vi "Install Linux Image.vi"(8 "error in (no error)":errorcluster, 11 "Selected Targets":T1[](array[typedef]) {"Primary NIC"."IP Address Request Mode" items=["Static"=1, "DHCP/Link-Local"=2, "Link-Local Only"=4, "DHCP Only"=8]}) -> (0 "error out":errorcluster, 1 "Cancelled":bool)   [LabVIEW 2020]
uses:
  Controls/Installation Internal Variables.ctl
  Controls/Target Information.ctl
  Controls/Target Network Settings.ctl
  Controls/System Credentials.ctl
  Controls/Installation Notifiers.ctl
  Controls/Deployment Status Data Type.ctl
  Controls/Deployment Progress Data Type.ctl
  Controls/FP Control Functions.ctl
panel:
  out "Stop Updates":bool
  in  "Start Installation Process":bool
  in  "Stop":bool
  in  "Internal Variables":T4 {"Targets"."Primary NIC"."IP Address Request Mode" items=["Static"=1, "DHCP/Link-Local"=2, "Link-Local Only"=4, "DHCP Only"=8]}
  out "Targets":i32(listbox)
  in  "Close":bool
  # "Targets"
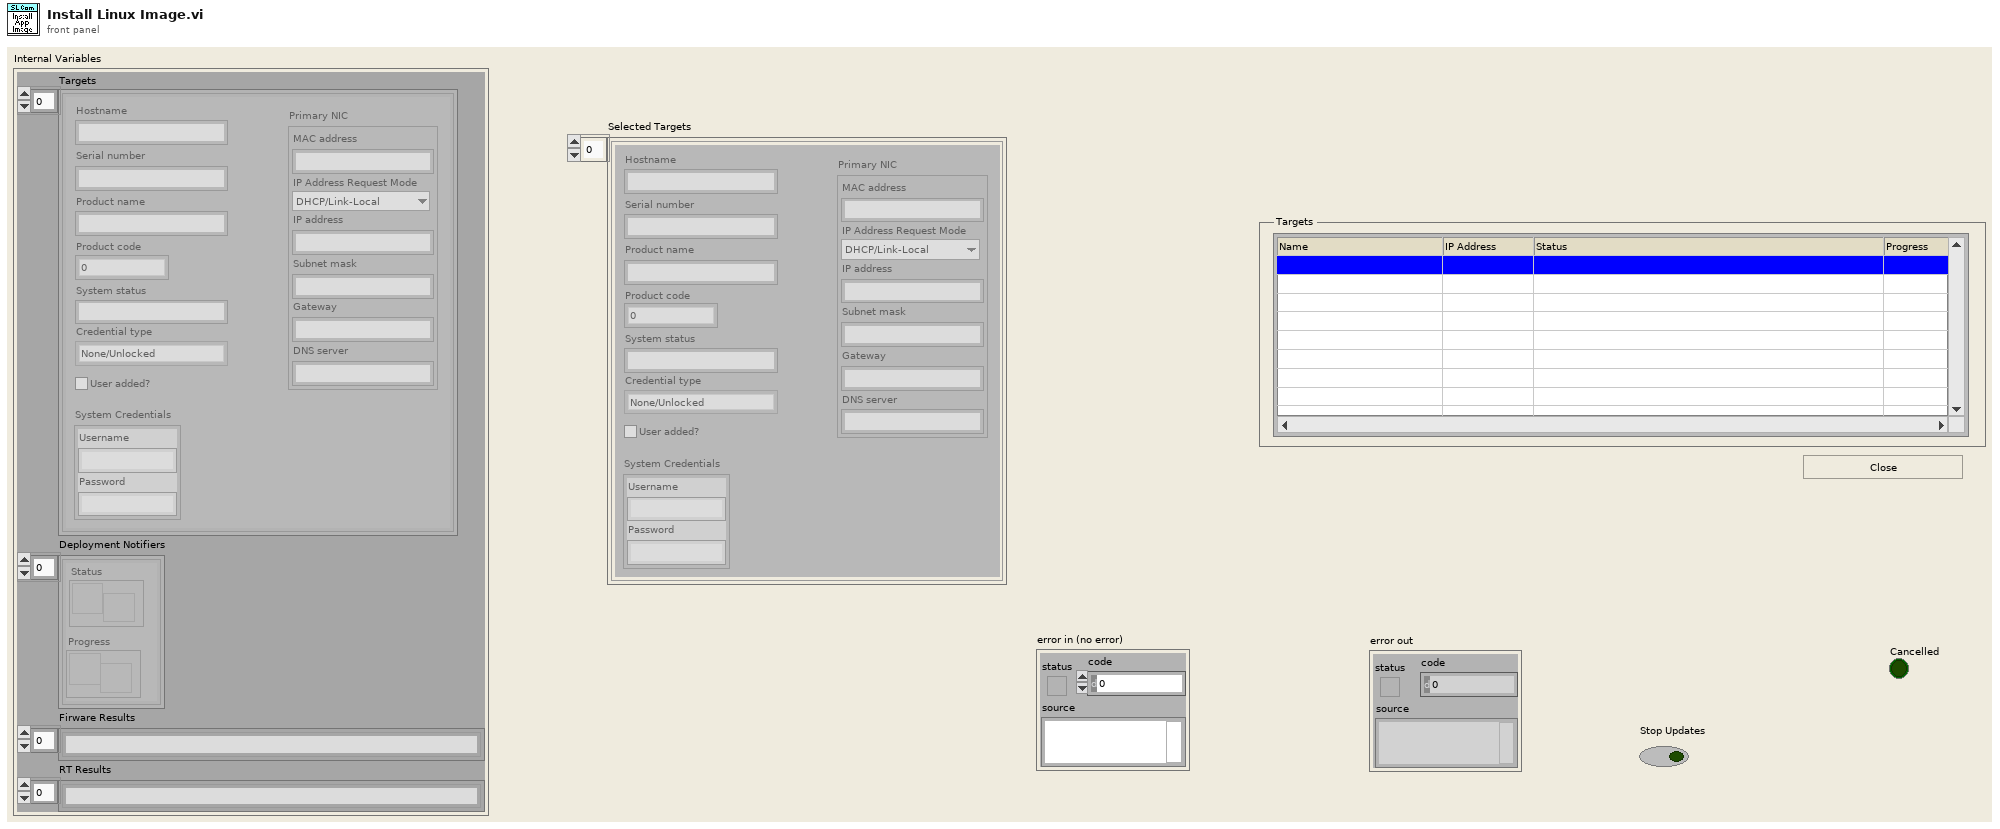
[diagram p1: front panel]
types:
  T1 = typedef "Target Information.ctl" = cluster{"Hostname":string, "Serial number":string, "Product name":string, "Product code":i32, "System status":string, "Credential type":enum16{"None/Unlocked", "FTP Password", "NIAuth Credentials"}, "User added?":bool, "Primary NIC":T2, "System Credentials":T3}
  T2 = typedef "Target Network Settings.ctl" = cluster{"MAC address":string, "IP Address Request Mode":i32, "IP address":string, "Subnet mask":string, "Gateway":string, "DNS server":string}
  T3 = typedef "System Credentials.ctl" = cluster{"Username":string, "Password":string}
  T4 = typedef "Installation Internal Variables.ctl" = cluster{"Targets":T1[], "Deployment Notifiers":T5[], "Firware Results":string[], "RT Results":string[]}
  T5 = typedef "Installation Notifiers.ctl" = cluster{"Status":refnum<notifier>, "Progress":refnum<notifier>}
  T6 = enum8{"Enabled", "Disabled", "Disabled and Grayed Out"}
  T7 = typedef "Deployment Progress Data Type.ctl" = i8
  T8 = typedef "Deployment Status Data Type.ctl" = string
  T9 = typedef "FP Control Functions.ctl" = enum16{"Open", "Close", "Bring To Front", "Center"}
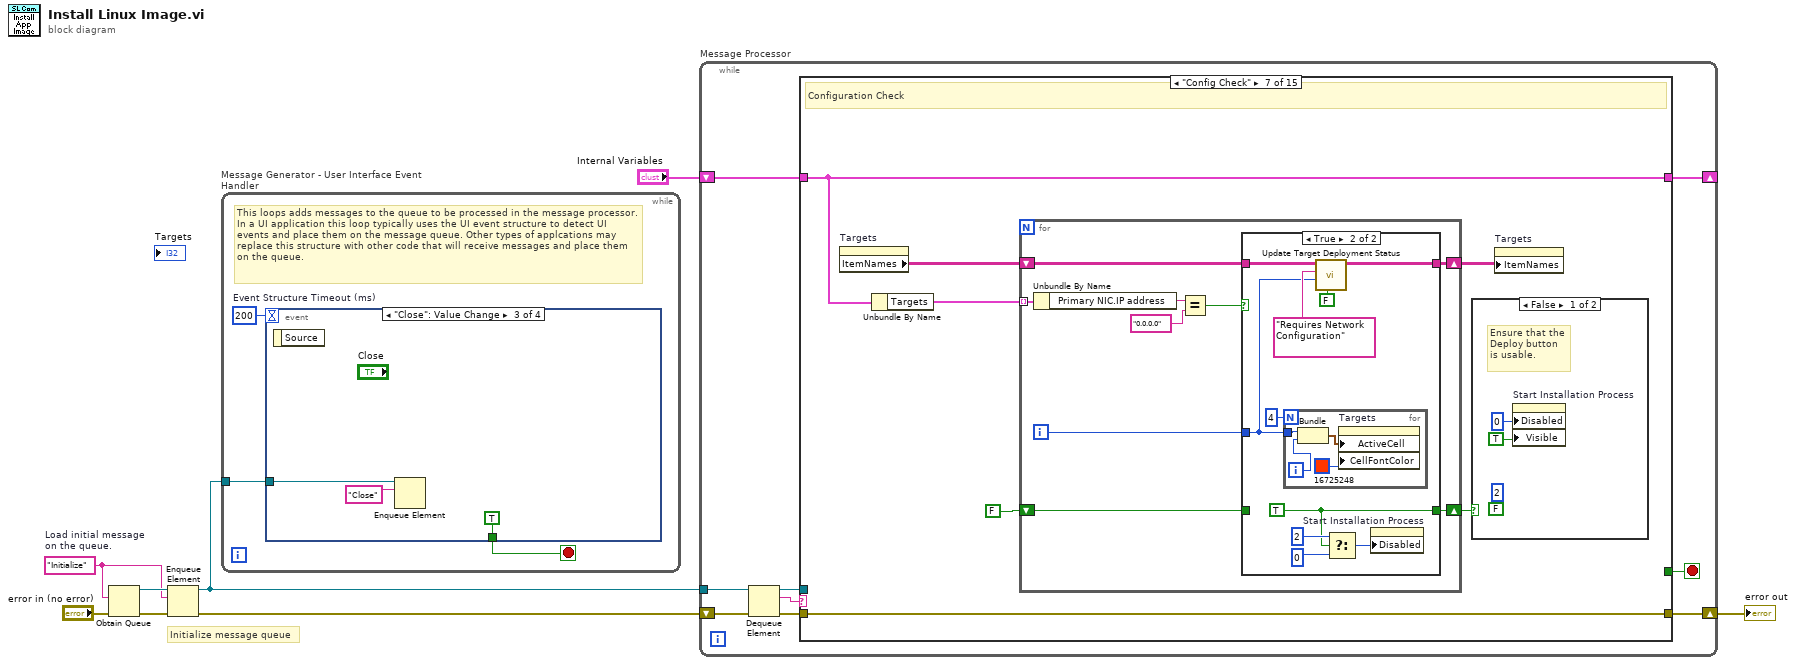
[diagram p0: block diagram]
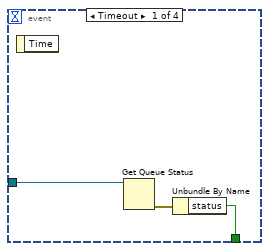
[diagram p2: hidden frame]
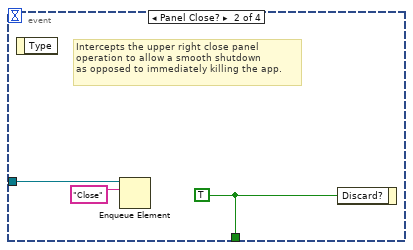
[diagram p3: hidden frame]
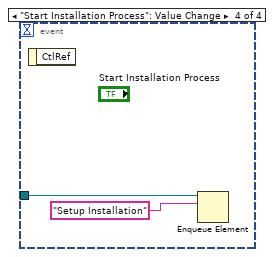
[diagram p4: hidden frame]
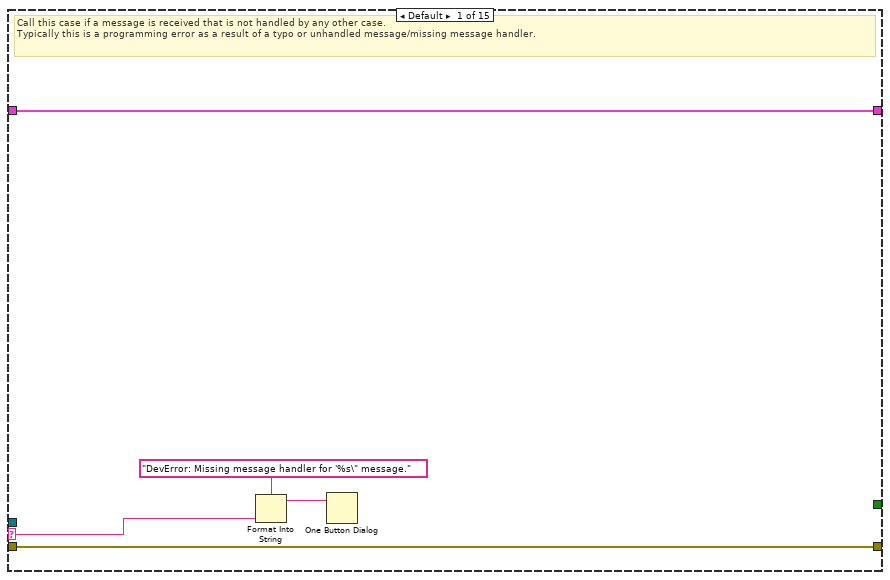
[diagram p5: hidden frame]
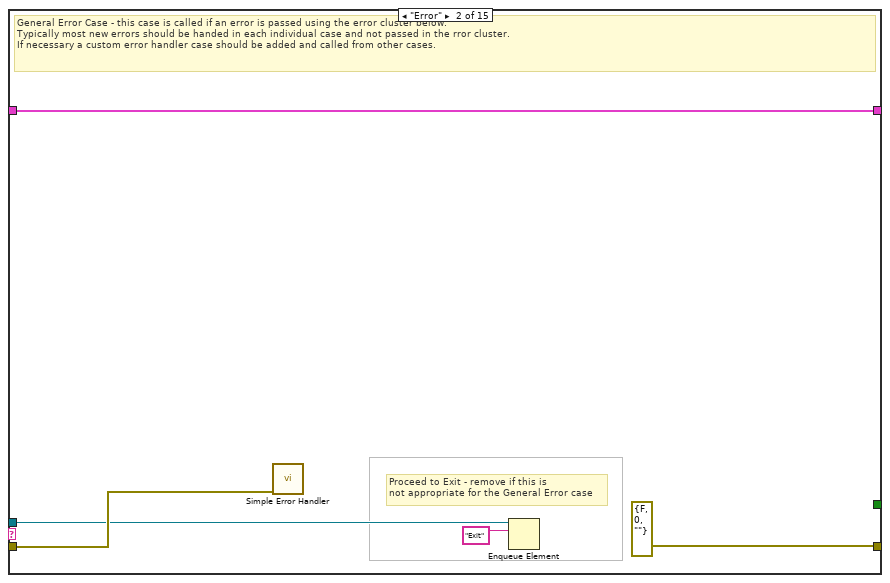
[diagram p6: hidden frame]
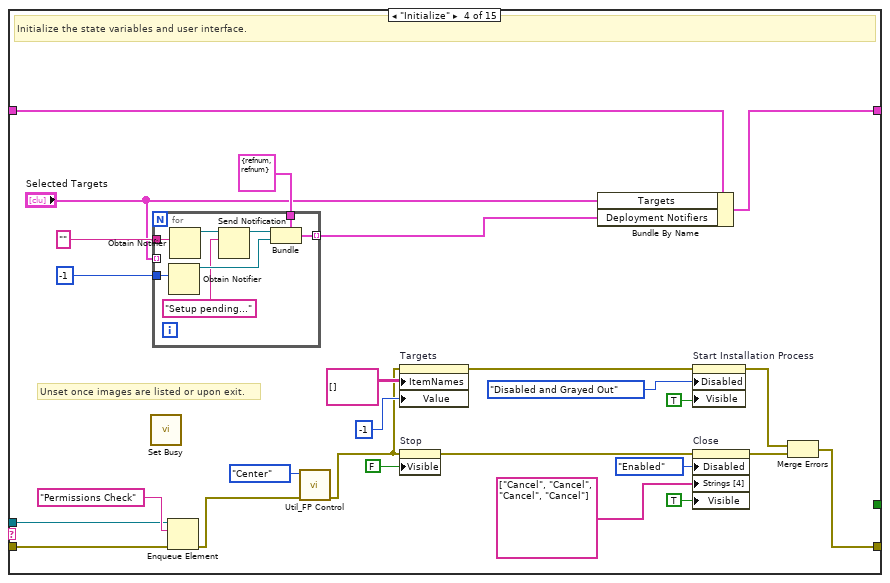
[diagram p8: hidden frame]
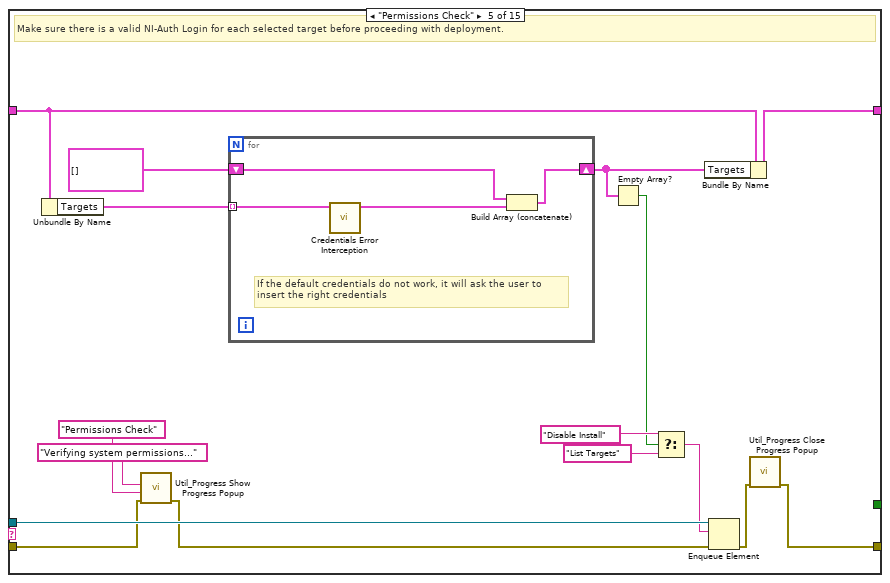
[diagram p9: hidden frame]
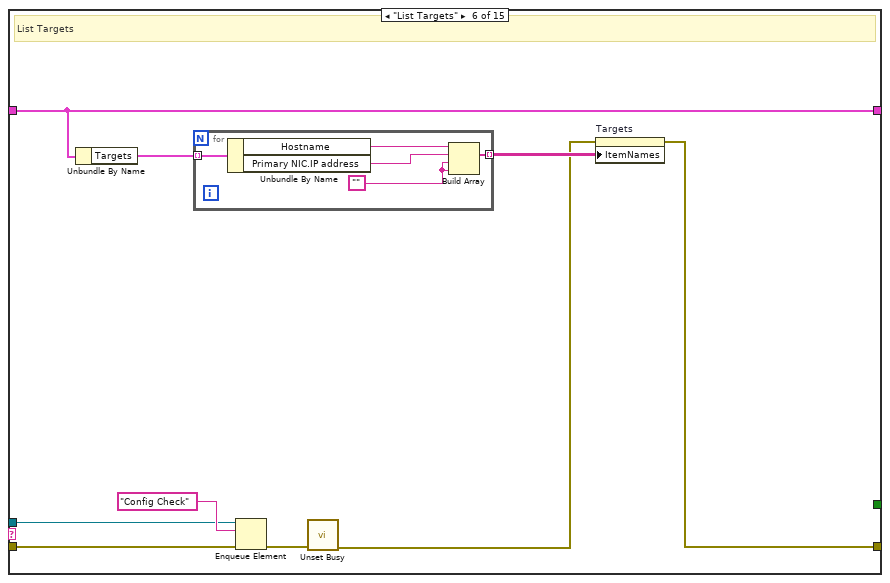
[diagram p10: hidden frame]
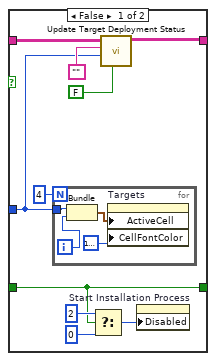
[diagram p12: hidden frame]
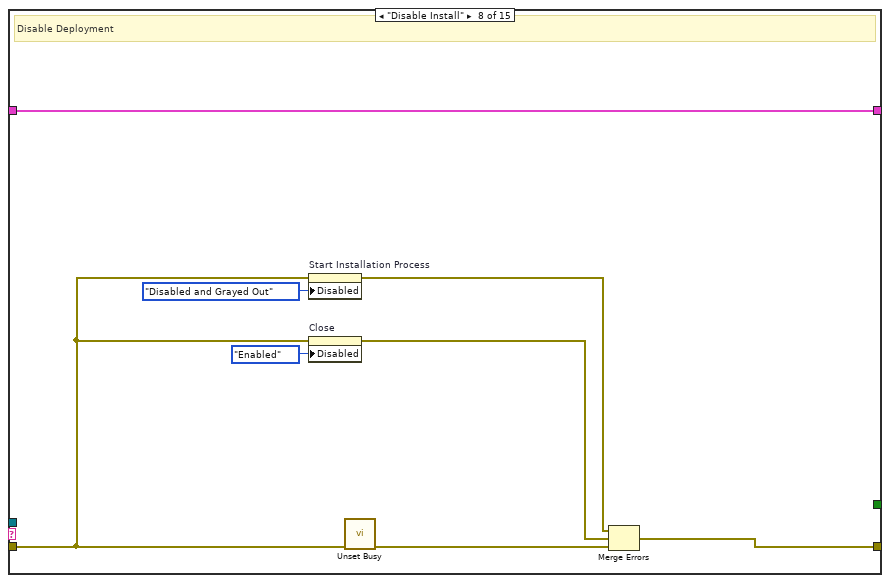
[diagram p13: hidden frame]
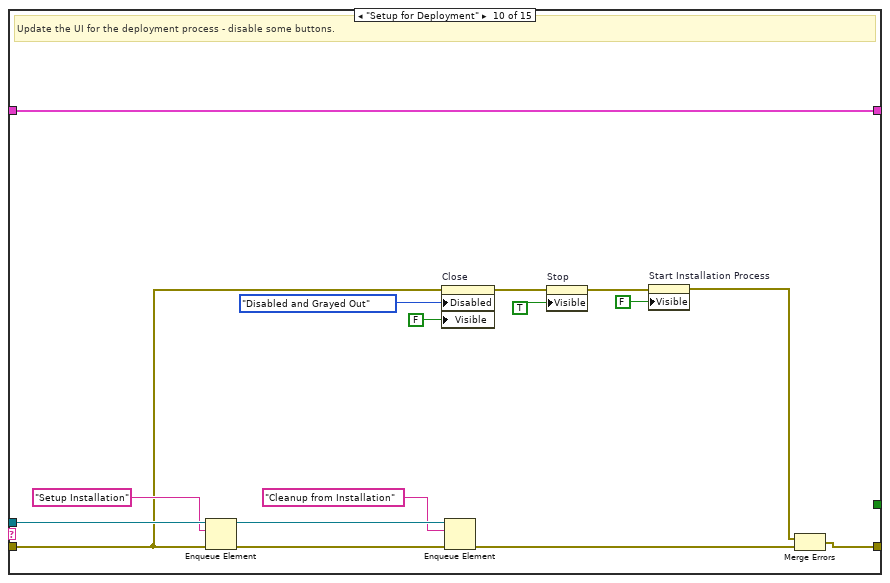
[diagram p15: hidden frame]
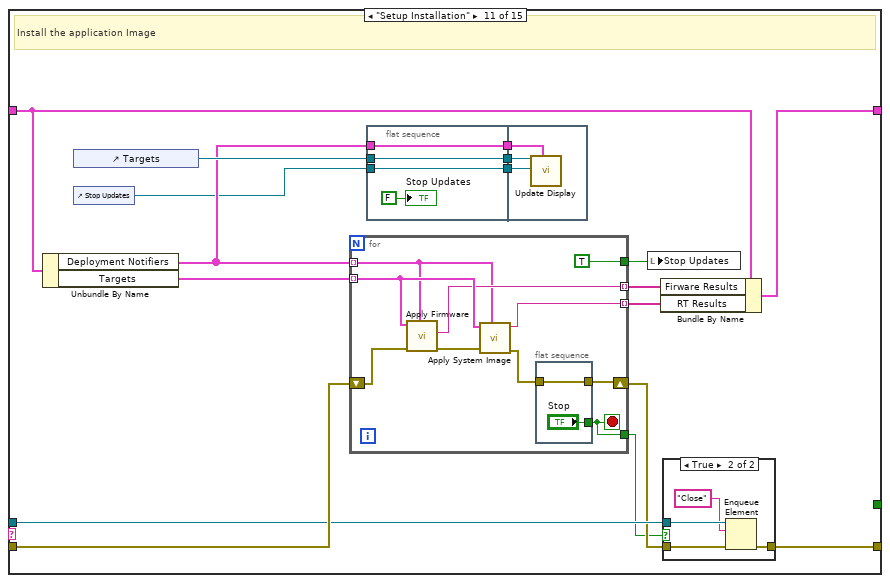
[diagram p16: hidden frame]
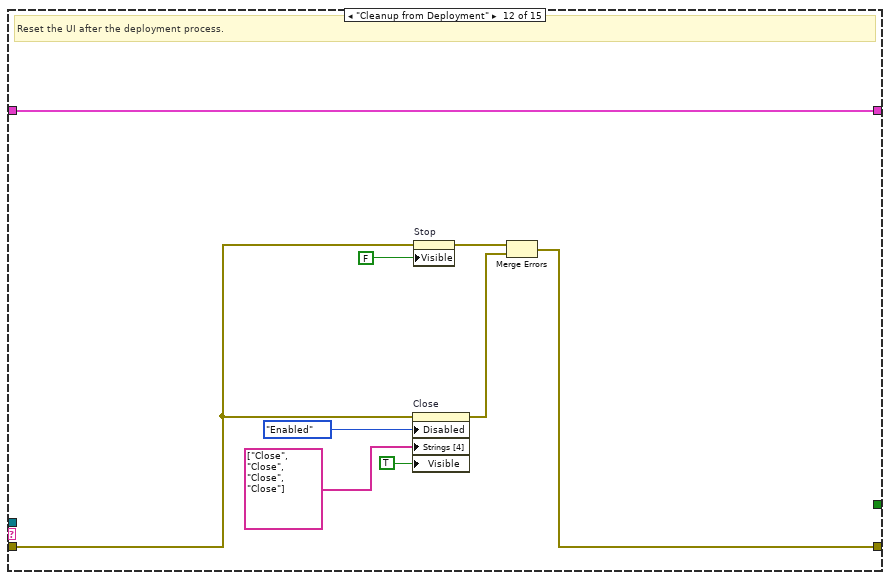
[diagram p18: hidden frame]
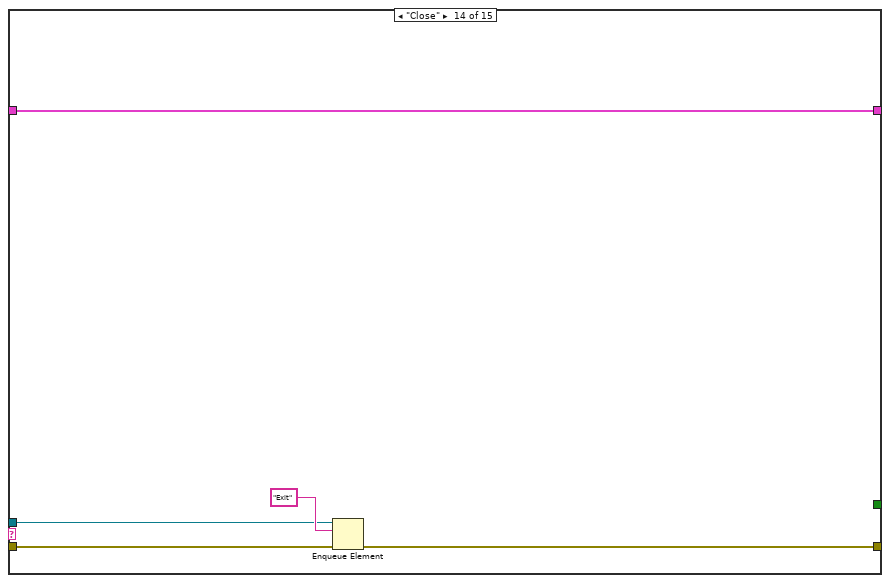
[diagram p20: hidden frame]
diagram:
  w1 = "Initialize"  # Load initial message on the queue.
  # "Initialize message queue"
  n1 = Obtain Queue(element data type=w1, error in (no error)="error in (no error)") -> (queue out=w3:refnum<queue>, error out=w8:errorcluster)  [unwired: 3 in, 1 out]
  n2 = Enqueue Element(queue=w3, element=w1, error in (no error)=w8) -> (queue out=w2:refnum<queue>, error out=w4:errorcluster)  [unwired: 1 in, 1 out]
  n3 = while "Message Generator - User Interface Event Handler" {
    tunnel: w2 -> [w9]
    stop <- w10 stop-if-true
    w11 = 200  # Event Structure Timeout (ms)
    # "This loops adds messages to the queue to be processed in the message processor. In a UI application this loop typically uses the UI event structure to detect UI events and place them on the message queue. Other types of applcations may replace this structure with other code that will receive messages and place them on the queue."
    n4 = event shown="[2] \"Close\": Value Change" {
      selector: _ -> [_ _ _ _]
      dyn-events: _ -> [_ _ _ _]
      timeout: w11 -> [_ _ _ _]
      tunnel: [w13 w17 TRUE ("Discard?") _] -> w10
      tunnel: w9 -> [w12 w16 w20 w22]
      event Timeout {
        n5 = event-data() -> ()  [unwired: 2 out]
        n6 = Get Queue Status(queue=w12) -> (error out=w14:errorcluster)  [unwired: 2 in, 7 out]
        n7 = Unbundle By Name(w14) -> ("status"=w13:bool)
      }
      event Panel Close? {
        w17 = TRUE ("Discard?")
        # "Intercepts the upper right close panel\noperation to allow a smooth shutdown\nas opposed to immediately killing the app."
        n8 = event-data() -> ()  [unwired: 2 out]
        n9 = Enqueue Element(queue=w16, element="Close") -> ()  [unwired: 2 in, 3 out]
        n10 = event-data("Discard?"=w17) -> ()  [unwired: 1 in, 1 out]
      }
      event "Close": Value Change {
        n11 = event-data() -> ()  [unwired: 2 out]
        n12 = Enqueue Element(queue=w20, element="Close") -> ()  [unwired: 2 in, 3 out]
      }
      event "Start Installation Process": Value Change {
        n13 = event-data() -> ()  [unwired: 2 out]
        n14 = Enqueue Element(queue=w22, element="Setup Installation") -> ()  [unwired: 2 in, 3 out]
      }
    }
  }
  n15 = while "Message Processor" {
    shift-left: w4 -> [w26]
    shift-right: [w27] -> w5
    tunnel: w2 -> [w25]
    shift-left: "Internal Variables" -> [w31]
    shift-right: [w30] -> _
    stop <- w23 stop-if-true
    n16 = Dequeue Element(queue=w25, error in (no error)=w26) -> (queue out=w29:refnum<queue>, element=w24:string, error out=w28:errorcluster)  [unwired: 1 in, 1 out]
    n17 = case shown="\"Config Check\"" w24 {
      selector: w24 -> [w34 _ _ _ _ _ _ _ _ _ _ _ _ _ _]
      tunnel: [w36 w41 w43 w68 w90 w104 w114 w164 w167 w183 w187 w232 w235 w240 w246] -> w30
      tunnel: w31 -> [w36 w41 w43 w69 w91 w104 w114 w164 w167 w183 w200 w232 w235 w240 w246]
      tunnel: w29 -> [_ w38 _ w57 w89 w101 _ _ _ w179 w198 _ _ w237 w251]
      tunnel: w28 -> [w35 w39 w42 w63 w85 w102 w118 w161 w166 w172 w199 w228 w234 w238 w252]
      tunnel: [w35 errorcluster {"status"=FALSE, "code"=0, "source"=""} ("error out") w42 w45 w79 w98 w118 w160 w166 w169 w196 w225 w234 w236 w243] -> w27
      tunnel: [_ _ _ _ _ _ _ _ _ _ _ _ _ _ TRUE] -> w23
      frame Default {
        # "Call this case if a message is received that is not handled by any other case.\nTypically this is a programming error as a result of a typo or unhandled message/missing message handler."
        n18 = Format Into String(format string="DevError: Missing message handler for '%s\" message." ("message"), w34) -> (resulting string=w32:string)  [unwired: 2 in, 1 out]
        n19 = One Button Dialog(message=w32) -> ()  [unwired: 2 out]
      }
      frame "Error" {
        # "Proceed to Exit - remove if this is\nnot appropriate for the General Error case"
        # "General Error Case - this case is called if an error is passed using the error cluster below.\nTypically most new errors should be handed in each individual case and not passed in the rror cluster.\nIf necessary a custom error handler case should be added and called from other cases."
        n20 = call <vilib>:"Simple Error Handler.vi"("error in (no error)"=w39) -> ()  [unwired: 1 in, 8 out]
        n21 = Enqueue Element(queue=w38, element="Exit") -> ()  [unwired: 2 in, 3 out]
      }
      frame "*******Init******" {
        # "Dummy case to add a seperator in the Case Structure menu."
      }
      frame "Initialize" {
        # "Unset once images are listed or upon exit."
        # "Initialize the state variables and user interface."
        n22 = call <vilib>:"Set Busy.vi"() -> ()  [unwired: 10 in, 2 out]
        n23 = for {
          tunnel: T8 "" ("status notifier data type") -> [w77]
          tunnel: T7 -1 ("Progress") -> [w76]
          tunnel: T5 {"Status"=refnum, "Progress"=refnum} ("Deployment Notifiers") -> [w74]
          tunnel: [w73] -> w59 mode=indexing
          tunnel: "Selected Targets" -> [_] mode=indexing
          n24 = Obtain Notifier(notification data type=w76) -> (notifier out=w75:refnum<notifier>)  [unwired: 3 in, 2 out]
          n25 = Obtain Notifier(notification data type=w77) -> (notifier out=w72:refnum<notifier>)  [unwired: 3 in, 2 out]
          n26 = Send Notification(notification=T8 "Setup pending...", notifier=w72) -> (notifier out=w71:refnum<notifier>)  [unwired: 1 in, 1 out]
          n27 = Bundle(cluster=w74, "Status"=w71, "Progress"=w75) -> (w73:T5)
        }
        n28 = Enqueue Element(queue=w57, element="Permissions Check", error in (no error)=w63) -> (error out=w51:errorcluster)  [unwired: 1 in, 2 out]
        n29 = call "Util_FP Control.vi"("error in (no error)"=w51, "Function"=FP_Control_Functions."Center") -> ("error out"=w50:errorcluster)  [unwired: 9 out]
        n30 = property on="Targets" class="MCListbox (strict)"(error in=w50, "ItemNames"=string[][] [] ("Item Names"), "Value"=-1 ("Targets")) -> (error out=w49:errorcluster)  [unwired: 1 in, 1 out]
        n31 = property on="Stop" class="Bool"(error in=w50, "Visible"=FALSE) -> (error out=w48:errorcluster)  [unwired: 1 in, 1 out]
        n32 = Bundle By Name(cluster=w69, "Targets"="Selected Targets", "Deployment Notifiers"=w59) -> (w68:T4)
        n33 = property on="Start Installation Process" class="Bool"(error in=w49, "Disabled"=T6."Disabled and Grayed Out", "Visible"=TRUE) -> (error out=w47:errorcluster)  [unwired: 1 in, 1 out]
        n34 = property on="Close" class="Bool"(error in=w48, "Disabled"=T6."Enabled", "Strings [4]"=string[] ["Cancel", "Cancel", "Cancel", "Cancel"], "Visible"=TRUE) -> (error out=w46:errorcluster)  [unwired: 1 in, 1 out]
        n35 = Merge Errors(w47, w46) -> (w45:errorcluster)
      }
      frame "Permissions Check" {
        # "Make sure there is a valid NI-Auth Login for each selected target before proceeding with deployment."
        n36 = Unbundle By Name(w91) -> ("Targets"=w93:T1[])
        n37 = call "Util_Progress Show Progress Popup.vi"("error in (no error)"=w85, "Title"="Permissions Check" ("Message"), "Message"="Verifying system permissions...") -> ("error out"=w78:errorcluster)  [unwired: 8 in]
        n38 = for {
          tunnel: w93 -> [w95] mode=indexing
          shift-right: [w97] -> w81
          shift-left: T1[] [] -> [w96]
          # "If the default credentials do not work, it will ask the user to \ninsert the right credentials"
          n39 = call "Credentials Error Interception.vi"("Target settings in"=w95) -> ("Target settings out"=w94:T1)  [unwired: 9 in, 1 out]
          n40 = Build Array (concatenate)(w96, w94) -> (w97:T1[])
        }
        n41 = Empty Array?(array=w81) -> (empty?=w80:bool)
        n42 = Select(t="Disable Install", s=w80, f="List Targets") -> (s? t:f=w86:string)
        n43 = Bundle By Name(cluster=w91, "Targets"=w81) -> (w90:T4)
        n44 = Enqueue Element(queue=w89, element=w86, error in (no error)=w78) -> (error out=w84:errorcluster)  [unwired: 1 in, 2 out]
        n45 = call "Util_Progress Close Progress Popup.vi"("error in (no error)"=w84) -> ("error out"=w79:errorcluster)  [unwired: 10 in]
      }
      frame "List Targets" {
        # "List Targets"
        n46 = Unbundle By Name(w104) -> ("Targets"=w106:T1[])
        n47 = for {
          tunnel: w106 -> [w111] mode=indexing
          tunnel: [w108] -> w105 mode=indexing
          w107 = ""
          n48 = Unbundle By Name(w111) -> ("Hostname"=w110:string, "Primary NIC.IP address"=w109:string)
          n49 = Build Array(w110, w109, w107, w107) -> (w108:string[])
        }
        n50 = Enqueue Element(queue=w101, element="Config Check", error in (no error)=w102) -> (error out=w100:errorcluster)  [unwired: 1 in, 2 out]
        n51 = call <vilib>:"Unset Busy.vi"("error in (no error)"=w100) -> ("error out"=w99:errorcluster)  [unwired: 10 in]
        n52 = property on="Targets" class="MCListbox (strict)"(error in=w99, "ItemNames"=w105) -> (error out=w98:errorcluster)  [unwired: 1 in, 1 out]
      }
      frame "Config Check" {
        # "Configuration Check"
        n53 = property on="Targets" class="MCListbox (strict)"() -> ("ItemNames"=w113:string[][])  [unwired: 2 in, 2 out]
        n54 = Unbundle By Name(w114) -> ("Targets"=w117:T1[])
        n55 = for {
          tunnel: w117 -> [w125] mode=indexing
          shift-right: [w122] -> w112
          shift-left: FALSE -> [w123]
          shift-right: [w127] -> w115
          shift-left: w113 -> [w124]
          i -> [w126]
          n56 = Unbundle By Name(w125) -> ("Primary NIC.IP address"=w129:string)
          n57 = Equal?(x=w129, y="0.0.0.0") -> (x = y?=w121:bool)
          n58 = case shown="True" w121 {
            tunnel: [w138 w153] -> w127
            tunnel: w126 -> [w136 w149]
            tunnel: w124 -> [w139 w150]
            tunnel: w123 -> [w131 _]
            tunnel: [w131 w147] -> w122
            frame False {
              n59 = for {
                N: 4 -> [_]
                tunnel: w136 -> [w142]
                i -> [w141]
                n60 = Bundle(w142, w141) -> (w140:cluster{i32, i32})  [unwired: 1 in]
                n61 = property on="Targets" class="MCListbox (strict)"("ActiveCell"=w140, "CellFontColor"=u32 16777222) -> ()  [unwired: 2 in, 2 out]
              }
              n62 = Select(t=2, s=w131, f=0) -> (s? t:f=w132:i32)
              n63 = call "Update Target Deployment Status.vi"("Add Timestamp?"=FALSE, "Target Index"=w136, "Message"="", "Targets Deployment Status"=w139) -> ("Targets Deployment Status"=w138:string[][])  [unwired: 7 in]
              n64 = property on="Start Installation Process" class="Bool"("Disabled"=w132) -> ()  [unwired: 2 in, 2 out]
            }
            frame True {
              w147 = TRUE
              n65 = for {
                N: 4 -> [_]
                tunnel: w149 -> [w156]
                i -> [w155]
                n66 = Bundle(w156, w155) -> (w154:cluster{i32, i32})  [unwired: 1 in]
                n67 = property on="Targets" class="MCListbox (strict)"("ActiveCell"=w154, "CellFontColor"=u32 16725248) -> ()  [unwired: 2 in, 2 out]
              }
              n68 = call "Update Target Deployment Status.vi"("Add Timestamp?"=FALSE, "Target Index"=w149, "Message"="Requires Network Configuration", "Targets Deployment Status"=w150) -> ("Targets Deployment Status"=w153:string[][])  [unwired: 7 in]
              n69 = Select(t=2, s=w147, f=0) -> (s? t:f=w146:i32)
              n70 = property on="Start Installation Process" class="Bool"("Disabled"=w146) -> ()  [unwired: 2 in, 2 out]
            }
          }
        }
        n71 = case shown="False" w112 {
          frame False {
            (unwired) 2
            (unwired) FALSE ("Visible")
            # "Ensure that the\nDeploy button\nis usable."
            n72 = property on="Start Installation Process" class="Bool"("Disabled"=0, "Visible"=TRUE) -> ()  [unwired: 2 in, 2 out]
          }
          frame True {
          }
        }
        n73 = property on="Targets" class="MCListbox (strict)"("ItemNames"=w115) -> ()  [unwired: 2 in, 2 out]
      }
      frame "Disable Install" {
        # "Disable Deployment"
        n74 = property on="Start Installation Process" class="Bool"(error in=w161, "Disabled"=T6."Disabled and Grayed Out") -> (error out=w159:errorcluster)  [unwired: 1 in, 1 out]
        n75 = property on="Close" class="Bool"(error in=w161, "Disabled"=T6."Enabled") -> (error out=w158:errorcluster)  [unwired: 1 in, 1 out]
        n76 = call <vilib>:"Unset Busy.vi"("error in (no error)"=w161) -> ("error out"=w165:errorcluster)  [unwired: 10 in]
        n77 = Merge Errors(w159, w158, w165) -> (w160:errorcluster)
      }
      frame "*****************" {
        # "Dummy case to add a seperator in the Case Structure menu."
      }
      frame "Setup for Deployment" {
        # "Update the UI for the deployment process - disable some buttons."
        n78 = Enqueue Element(queue=w179, element="Setup Installation", error in (no error)=w172) -> (queue out=w176:refnum<queue>, error out=w177:errorcluster)  [unwired: 1 in, 1 out]
        n79 = property on="Close" class="Bool"(error in=w172, "Disabled"=T6."Disabled and Grayed Out", "Visible"=FALSE) -> (error out=w171:errorcluster)  [unwired: 1 in, 1 out]
        n80 = Enqueue Element(queue=w176, element="Cleanup from Installation", error in (no error)=w177) -> (error out=w175:errorcluster)  [unwired: 1 in, 2 out]
        n81 = property on="Stop" class="Bool"(error in=w171, "Visible"=TRUE) -> (error out=w170:errorcluster)  [unwired: 1 in, 1 out]
        n82 = property on="Start Installation Process" class="Bool"(error in=w170, "Visible"=FALSE) -> (error out=w168:errorcluster)  [unwired: 1 in, 1 out]
        n83 = Merge Errors(w168, w175) -> (w169:errorcluster)
      }
      frame "Setup Installation" {
        # "Install the application Image"
        n84 = Unbundle By Name(w200) -> ("Deployment Notifiers"=w194:T5[], "Targets"=w188:T1[])
        n85 = control-ref of="Targets"() -> (w195:refnum<vi>)
        n86 = control-ref of="Stop Updates"() -> (w190:refnum<vi>)
        n87 = for {
          shift-right: [w217] -> w197
          shift-left: w199 -> [w220]
          tunnel: [w222] -> w184
          tunnel: w194 -> [w213] mode=indexing
          tunnel: [TRUE] -> w193
          tunnel: w188 -> [w216] mode=indexing
          tunnel: [w215] -> w186 mode=indexing
          tunnel: [w214] -> w185 mode=indexing
          stop <- w222 stop-if-true
          n88 = call "Apply Firmware.vi"("Installation Notifiers"=w213, "error in"=w220, "Target settings"=w216) -> ("error out"=w219:errorcluster, "Detailed Result"=w215:string)  [unwired: 6 in, 1 out]
          n89 = call "Apply System Image.vi"("Installation Notifiers"=w213, "error in"=w219, "Target settings"=w216) -> ("error out"=w218:errorcluster, "Real-Time:System Status"=w214:string)  [unwired: 7 in]
          n90 = flat-sequence {
            tunnel: ["Stop"] -> w222
            tunnel: w218 -> [w223]
            tunnel: [w223] -> w217
            frame #0 {
            }
          }
        }
        n91 = flat-sequence {
          tunnel: w194 -> [w203]
          tunnel: w195 -> [w204]
          tunnel: [w204] -> w192
          tunnel: [w203] -> w191
          tunnel: w190 -> [w202]
          tunnel: [w202] -> w189
          tunnel: w192 -> [w207]
          tunnel: w191 -> [w206]
          tunnel: w189 -> [w205]
          frame #0 {
            "Stop Updates" <- FALSE ("Stop Updates")
          }
          frame #1 {
            n92 = call "Update Display.vi"("Deployment Notifiers"=w206, "Stop Updates"=w205, "Listbox Reference"=w207) -> ()  [unwired: 9 in]
          }
        }
        n93 = local write "Stop Updates"(w193) -> ()
        n94 = Bundle By Name(cluster=w200, "Firware Results"=w186, "RT Results"=w185) -> (w187:T4)
        n95 = case shown="True" w184 {
          tunnel: w198 -> [_ w212]
          tunnel: w197 -> [w208 w211]
          tunnel: [w208 w210] -> w196
          frame False {
          }
          frame True {
            n96 = Enqueue Element(queue=w212, element="Close" ("Message Name"), error in (no error)=w211) -> (error out=w210:errorcluster)  [unwired: 1 in, 2 out]
          }
        }
      }
      frame "Cleanup from Deployment" {
        # "Reset the UI after the deployment process."
        n97 = property on="Close" class="Bool"(error in=w228, "Disabled"=T6."Enabled", "Strings [4]"=string[] ["Close", "Close", "Close", "Close"], "Visible"=TRUE) -> (error out=w226:errorcluster)  [unwired: 1 in, 1 out]
        n98 = property on="Stop" class="Bool"(error in=w228, "Visible"=FALSE) -> (error out=w227:errorcluster)  [unwired: 1 in, 1 out]
        n99 = Merge Errors(w227, w226) -> (w225:errorcluster)
      }
      frame "******Close******" {
        # "Dummy case to add a seperator in the Case Structure menu."
      }
      frame "Close" {
        n100 = Enqueue Element(queue=w237, element="Exit", error in (no error)=w238) -> (error out=w236:errorcluster)  [unwired: 1 in, 2 out]
      }
      frame "Exit" {
        n101 = Unbundle By Name(w246) -> ("Deployment Notifiers"=w245:T5[])
        n102 = Release Queue(queue=w251, force destroy? (F)=TRUE, error in (no error)=w252) -> (error out=w244:errorcluster)  [unwired: 2 out]
        n103 = for {
          tunnel: w245 -> [w258] mode=indexing
          shift-right: [w253] -> w243
          shift-left: w244 -> [w256]
          n104 = Unbundle By Name(w258) -> ("Status"=w257:refnum<notifier>, "Progress"=w255:refnum<notifier>)
          n105 = Release Notifier(notifier=w257, force destroy? (F)=TRUE, error in (no error)=w256) -> (error out=w254:errorcluster)  [unwired: 2 out]
          n106 = Release Notifier(notifier=w255, force destroy? (F)=TRUE, error in (no error)=w254) -> (error out=w253:errorcluster)  [unwired: 2 out]
        }
        n107 = property on="Close" class="Bool"() -> ("Strings [4]"=w250:string[])  [unwired: 2 in, 2 out]
        n108 = Index Array(array=w250) -> (element=w249:string)  [unwired: 1 in]
        n109 = Equal?(x="Cancel", y=w249) -> (x = y?=→"Cancelled":bool)
        n110 = call <vilib>:"Unset Busy.vi"() -> ()  [unwired: 11 in, 1 out]
      }
    }
  }
  "error out" <- w5
